vi "Get Re from X using calibration data (single point).vi"(1 "Calibration data":T1, 2 "X":dbl) -> (0 "Re":dbl format="%#_9g")   [LabVIEW 2022 SP3]
doc: "Get Re = f(X) for a single point in X using the calibration data as a lookup table.\n(Monotonic) cubic spline interpolation.\nPN 05-NOV-23."
uses:
  Ctls/Calibration data.ctl
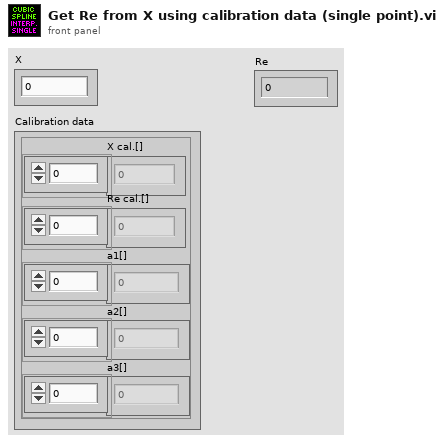
[diagram p1: front panel]
types:
  T1 = typedef "Calibration data.ctl" = cluster{"X cal.[]":dbl[], "Re cal.[]":dbl[], "a1[]":dbl[], "a2[]":dbl[], "a3[]":dbl[]}
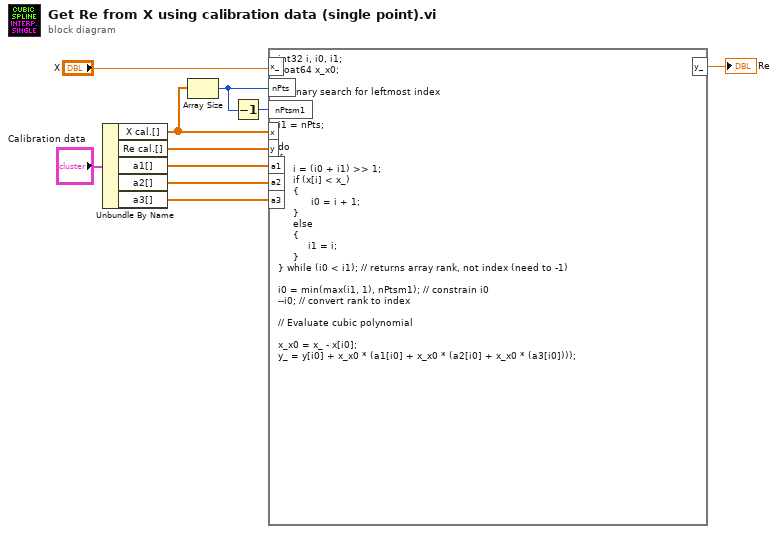
[diagram p0: block diagram]
diagram:
  n1 = Unbundle By Name("Calibration data") -> ("X cal.[]"=w2:dbl[], "Re cal.[]"=w1:dbl[], "a1[]"=w5:dbl[], "a2[]"=w4:dbl[], "a3[]"=w3:dbl[])
  n2 = Array Size(array=w2) -> (size(s)=w9:i32)
  n3 = Decrement(x=w9) -> (x-1=w7:i32)
  n4 = formula code="int32 i, i0, i1;\nfloat64 x_x0;\n\n// Binary search for leftmost index\n\ni0 = 0;\ni1 = nPts;\n\ndo\n{\n     i = (i0 + i1) >> 1;\n     if (x[i] < x_)\n     {\n           i0 = i + 1;\n     }\n     else\n     {\n          i1 = i;\n     }\n} while (i0 < i1); // returns array rank, not index (need to -1)\n\ni0 = min(max(i1, 1), nPtsm1); // constrain i0\n--i0; // convert rank to index\n\n// Evaluate cubic polynomial\n\nx_x0 = x_ - x[i0];\ny_ = y[i0] + x_x0 * (a1[i0] + x_x0 * (a2[i0] + x_x0 * (a3[i0])));"("x"=w2, "nPts"=w9, "x_"="X", "y"=w1, "nPtsm1"=w7, "a1"=w5, "a2"=w4, "a3"=w3) -> ("y_"=→"Re":dbl)
